vi "Variant_to_String.vi"(8 "Error in":errorcluster, 11 "Value (in)":variant) -> (0 "Error out":errorcluster, 2 "Value (string)":string, 3 "Value (out)":string)   [LabVIEW 2012]
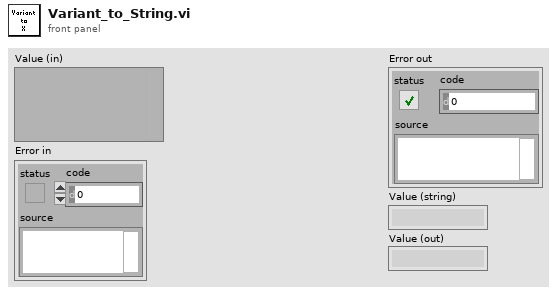
[diagram p1: front panel]
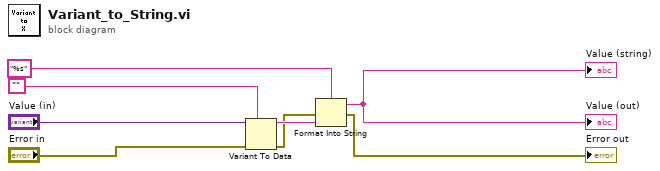
[diagram p0: block diagram]
diagram:
  n1 = Variant To Data(error in="Error in", type="", Variant="Value (in)") -> (data=w8:string, error out=w7:errorcluster)
  n2 = Format Into String(format string="%s", error in=w7, w8) -> (resulting string=→"Value (string)" →"Value (out)":string, error out=→"Error out":errorcluster)  [unwired: 1 in]
